vi "GOOP_GetClassProvider.vi"(1 "New Item Parent/Object":variant, 3 "CreateClass":bool, 5 "error in (no error)":errorcluster, 6 "ProviderClassType":T1) -> (15 "ProjectItem":refnum<vi>, 16 "LVClass.Open":refnum<vi>, 19 "error out":errorcluster)   [LabVIEW 2016]
uses:
  <resource>/Framework/Providers/Open_GDS/SubVIs/GOOP_ClassProviderClassType.ctl
  <resource>/Framework/Providers/API/mxLvNIIM.ctl
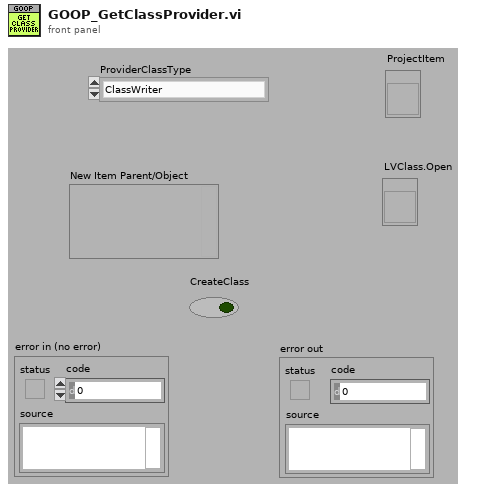
[diagram p1: front panel]
types:
  T1 = typedef "GOOP_ClassProviderClassType.ctl" = enum16{"ClassWriter", "ClassReader"}
  T2 = typedef "mxLvNIIM.ctl" = cluster{"Item URL":string, "Item ID":string, "Item Index":i32, "Specific Type":string}
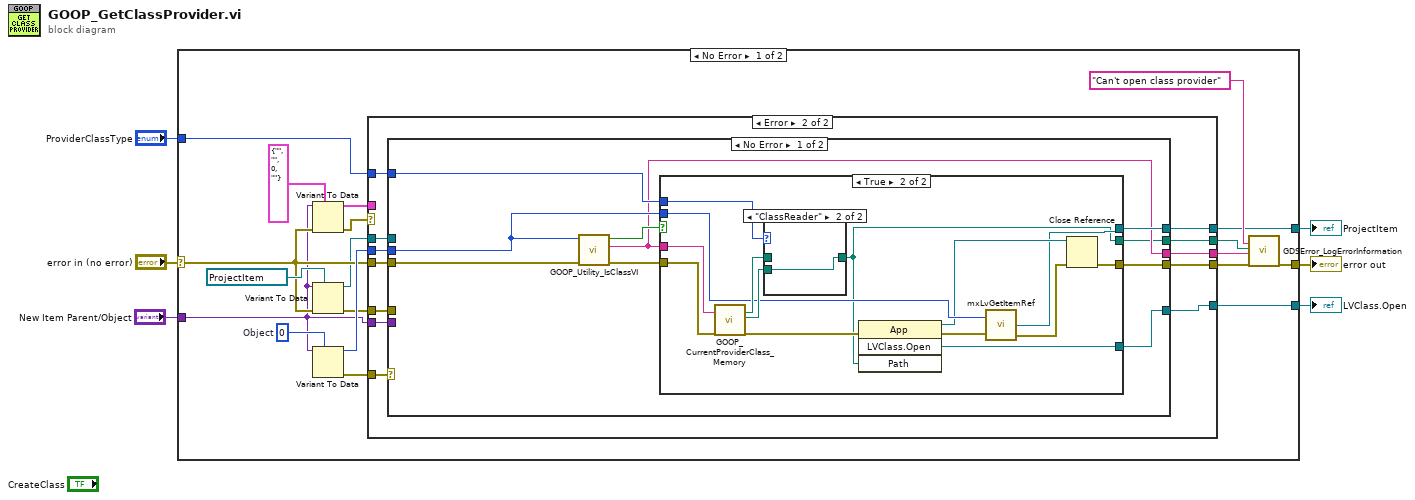
[diagram p0: block diagram]
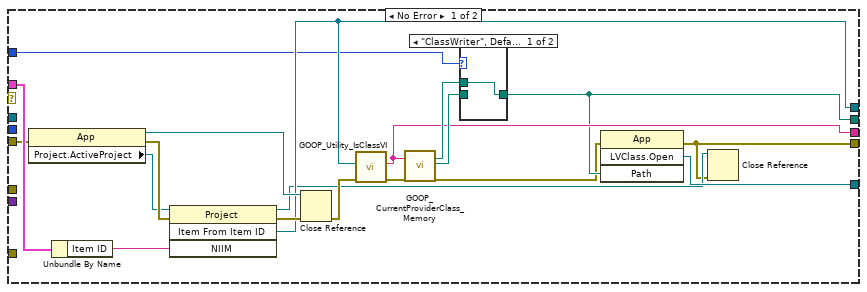
[diagram p2: hidden frame]
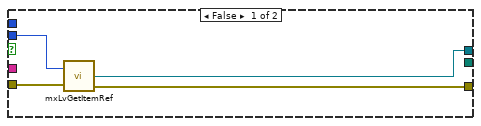
[diagram p4: hidden frame]
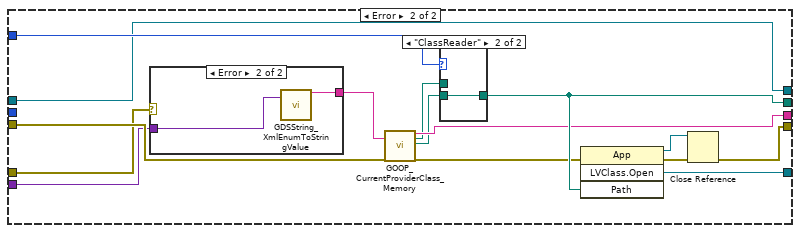
[diagram p6: hidden frame]
diagram:
  n1 = case shown="No Error" "error in (no error)" {
    selector: "error in (no error)" -> [w10 w108]
    tunnel: [w15 _] -> w2
    tunnel: [w13 _] -> w3
    tunnel: [w19 w108] -> w4
    tunnel: "New Item Parent/Object" -> [w7 _]
    tunnel: "ProviderClassType" -> [w20 _]
    frame No Error {
      w23 = u64 0  # Object
      n2 = Variant To Data(error in=w10, type=T2 {"Item URL"="", "Item ID"="", "Item Index"=0, "Specific Type"=""} ("New Item Parent"), Variant=w7) -> (data=w24:T2, error out=w21:errorcluster)
      n3 = Variant To Data(error in=w10, type=refnum<vi> refnum ("My Computer"), Variant=w7) -> (data=w8:refnum<vi>, error out=w9:errorcluster)
      n4 = Variant To Data(type=w23, Variant=w7) -> (data=w22:u64, error out=w12:errorcluster)  [unwired: 1 in]
      n5 = case shown="Error" w21 {
        tunnel: [w44 w54] -> w15
        tunnel: [w36 w55] -> w13
        tunnel: w10 -> [w26 w58]
        tunnel: [w28 w53] -> w18
        tunnel: w24 -> [w41 _]
        tunnel: w22 -> [_ w56]
        tunnel: w20 -> [w32 w57]
        tunnel: [w34 w52] -> w17
        tunnel: [w33 w51] -> w14
        tunnel: w12 -> [_ w50]
        tunnel: w9 -> [_ w49]
        tunnel: w8 -> [_ w48]
        tunnel: w7 -> [_ w47]
        frame No Error {
          n6 = property class="App"(error in=w26) -> (reference out=w42:refnum<vi>, error out=w40:errorcluster, "Project.ActiveProject"=w31:refnum<vi>)  [unwired: 1 in]
          n7 = Unbundle By Name(w41) -> ("Item ID"=w39:string)
          n8 = invoke class="Project" method="Item From Item ID"(reference=w31, error in=w40, "NIIM"=w39) -> (reference out=w29:refnum<vi>, error out=w43:errorcluster, "GetItemFromNIIM"=w36:refnum<vi>)  [unwired: 1 in, 1 out]
          n9 = Close Reference(reference=w42, error in (no error)=w43) -> (error out=w30:errorcluster)
          n10 = call <resource>:"GOOP_Utility_IsClassVI.vi"("error in (no error)"=w30, "ProjectItem"=w36) -> ("error out"=w35:errorcluster, "ClassProvider"=w34:string)  [unwired: 5 in, 3 out]
          n11 = call <resource>:"GOOP_CurrentProviderClass_Memory.vi"("GetThisClassProvidersPaths(Returns the default providor if not wired)"=w34, "error in (no error)"=w35) -> ("ClassProviderClassWriterPath"=w37:path, "ClassProviderClassReaderPath"=w38:path, "error out"=w27:errorcluster)  [unwired: 13 in, 2 out]
          n12 = case shown="\"ClassWriter\", Default" w32 {
            tunnel: w38 -> [_ w46]
            tunnel: [w45 w46] -> w33
            tunnel: w37 -> [w45 _]
            frame "ClassWriter", Default {
            }
            frame "ClassReader" {
            }
          }
          n13 = invoke class="App" method="LVClass.Open"(error in=w27, "Path"=w33) -> (error out=w28:errorcluster, "LVClass.Open"=w44:refnum<vi>)  [unwired: 2 in, 2 out]
          n14 = Close Reference(reference=w29, error in (no error)=w28) -> ()  [unwired: 1 out]
        }
        frame Error {
          n15 = case shown="No Error" w50 {
            tunnel: w58 -> [w68 w99]
            tunnel: w57 -> [w66 w103]
            tunnel: w56 -> [w65 _]
            tunnel: [w64 w92] -> w55
            tunnel: [w63 w102] -> w54
            tunnel: [w62 w101] -> w53
            tunnel: [w60 w98] -> w52
            tunnel: [w59 w100] -> w51
            tunnel: w49 -> [_ w89]
            tunnel: w48 -> [_ w92]
            tunnel: w47 -> [_ w91]
            frame No Error {
              n16 = call <resource>:"GOOP_Utility_IsClassVI.vi"("error in (no error)"=w68, "Object"=w65) -> ("error out"=w67:errorcluster, "ClassProvider"=w60:string, "Is Class VI?"=w61:bool)  [unwired: 5 in, 2 out]
              n17 = case shown="True" w61 {
                tunnel: w67 -> [w72 w84]
                tunnel: w60 -> [_ w83]
                tunnel: w66 -> [_ w81]
                tunnel: w65 -> [w70 w79]
                tunnel: [w69 w74] -> w64
                tunnel: [_ w75] -> w63
                tunnel: [w71 w76] -> w62
                tunnel: [_ w73] -> w59
                frame False {
                  n18 = call <resource>:"mxLvGetItemRef.vi"("Item"=w70, "error in"=w72) -> ("Item Refnum"=w69:refnum<vi>, "error out"=w71:errorcluster)  [unwired: 1 out]
                }
                frame True {
                  n19 = call <resource>:"GOOP_CurrentProviderClass_Memory.vi"("GetThisClassProvidersPaths(Returns the default providor if not wired)"=w83, "error in (no error)"=w84) -> ("ClassProviderClassWriterPath"=w85:path, "ClassProviderClassReaderPath"=w86:path, "error out"=w82:errorcluster)  [unwired: 13 in, 2 out]
                  n20 = case shown="\"ClassReader\"" w81 {
                    tunnel: w86 -> [_ w88]
                    tunnel: [w87 w88] -> w73
                    tunnel: w85 -> [w87 _]
                    frame "ClassWriter", Default {
                    }
                    frame "ClassReader" {
                    }
                  }
                  n21 = invoke class="App" method="LVClass.Open"(error in=w82, "Path"=w73) -> (reference out=w77:refnum<vi>, error out=w80:errorcluster, "LVClass.Open"=w75:refnum<vi>)  [unwired: 2 in, 1 out]
                  n22 = call <resource>:"mxLvGetItemRef.vi"("Item"=w79, "error in"=w80) -> ("Item Refnum"=w74:refnum<vi>, "error out"=w78:errorcluster)  [unwired: 1 out]
                  n23 = Close Reference(reference=w77, error in (no error)=w78) -> (error out=w76:errorcluster)
                }
              }
            }
            frame Error {
              n24 = case shown="Error" w89 {
                tunnel: w91 -> [_ w105]
                tunnel: [_ w104] -> w90
                frame No Error {
                }
                frame Error {
                  n25 = call <resource>:"GDSString_XmlEnumToStringValue.vi"("EnumVariantIn(used if String is Empty)"=w105) -> ("EnumValueOut(string)"=w104:string)  [unwired: 15 in, 3 out]
                }
              }
              n26 = call <resource>:"GOOP_CurrentProviderClass_Memory.vi"("GetThisClassProvidersPaths(Returns the default providor if not wired)"=w90, "error in (no error)"=w99) -> ("ClassProviderName"=w98:string, "ClassProviderClassWriterPath"=w96:path, "ClassProviderClassReaderPath"=w97:path, "error out"=w95:errorcluster)  [unwired: 13 in, 1 out]
              n27 = case shown="\"ClassReader\"" w103 {
                tunnel: w97 -> [_ w107]
                tunnel: [w106 w107] -> w100
                tunnel: w96 -> [w106 _]
                frame "ClassWriter", Default {
                }
                frame "ClassReader" {
                }
              }
              n28 = invoke class="App" method="LVClass.Open"(error in=w95, "Path"=w100) -> (reference out=w94:refnum<vi>, error out=w93:errorcluster, "LVClass.Open"=w102:refnum<vi>)  [unwired: 2 in, 1 out]
              n29 = Close Reference(reference=w94, error in (no error)=w93) -> (error out=w101:errorcluster)
            }
          }
        }
      }
      n30 = call <resource>:"GDSError_LogErrorInformation.vi"("State"="Can't open class provider", "LocalVariableData"=w14, "ExtraErrorInfo"=w17, "error in (no error)"=w18) -> ("error out"=w19:errorcluster)  [unwired: 15 in]
    }
    frame Error {
    }
  }
  "error out" <- w4
  "LVClass.Open" <- w2
  "ProjectItem" <- w3
